vi "Move Scope Stage.vi"(7 "ABS":bool, 8 "error in (no error)":errorcluster, 10 "Deltas":cluster{"X":i32, "Y":i32, "Z":i32}, 11 "Port":string) -> (0 "error out":errorcluster, 2 "Response":string, 3 "Port out":string)   [LabVIEW 2012, in "Sciscan Scope Daemon.lvlib"]
uses:
  Sciscan Scope Daemon.lvlib
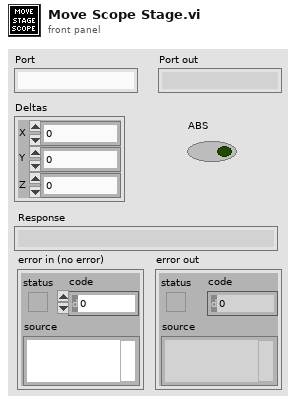
[diagram p1: front panel]
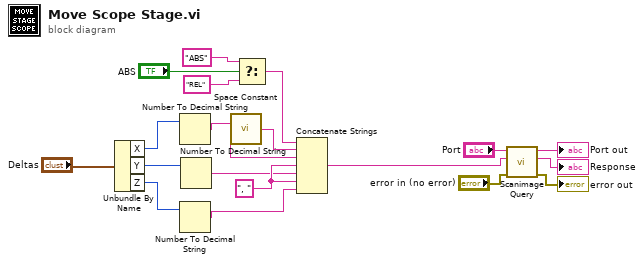
[diagram p0: block diagram]
diagram:
  w14 = ", " ("string")
  n1 = Unbundle By Name("Deltas") -> ("X"=w13:i32, "Y"=w12:i32, "Z"=w11:i32)
  n2 = Number To Decimal String(number=w13) -> (decimal integer string=w10:string)  [unwired: 1 in]
  n3 = Number To Decimal String(number=w11) -> (decimal integer string=w8:string)  [unwired: 1 in]
  n4 = Number To Decimal String(number=w12) -> (decimal integer string=w9:string)  [unwired: 1 in]
  n5 = call <vilib>:"Space Constant.vi"() -> ("String"=w15:string)
  n6 = Select(t="ABS", s="ABS", f="REL") -> (s? t:f=w16:string)
  n7 = Concatenate Strings(w16, w15, w10, w14, w9, w14, w8) -> (w3:string)
  n8 = call "Scanimage Query.vi"("error in"="error in (no error)", "query"=w3, "port"="Port") -> ("error out"=→"error out":errorcluster, "Response"=→"Response":string, "port out"=→"Port out":string)  [unwired: 6 in]
